vi "LakeShore Ramp Text In.vi"(1 "command text in":string[](array[string])=["N/A", "Magent PS", "N/A", "Set Field", "Set Field to 2.0000E+0 @ 0.0000T /min, no wait , extra 0 sec wait", "N/A", "N/A", "", "1", "0", "N/A", "2.000000", "0.000000", "N/A", "N/A", "N/A", "N/A", "N/A", "N/A", "N/A", "N/A", "N/A", "N/A", "N/A", "N/A", "N/A", "N/A", "N/A", "N/A", "N/A", "N/A", "N/A", "N/A", "N/A"]) -> (0 "LSRamp":T1={"VISA Resource Name"="", "extra wait"=0, "start (K/W)"=1e-09, "end (K/W)"=0.001, "Sweep Time (H:M:S)"=3600.0, "Mapping"=FALSE, "Parameter"=FALSE, "Loop"=FALSE} {"Sweep Time (H:M:S)" format="%<%H:%M:%S>t"; "extra wait" min=0; "start (K/W)" format="%#.7e"; "end (K/W)" format="%#.7e"})   [LabVIEW 2020]
uses:
  LSRamp.ctl
panel:
  # "LakeShore Ramp"
  # "Log"
  # "Start Temp(K)/Power(W)"
  # "Sweep Time (HH:MM:SS)"
  # "End Temp(K)/Power(W)"
  # "Linear"
  # "seconds"
  # "AND wait extra"
  # "Power"
  # "Temp"
  # "VISA Name"
  # "Loop 2"
  # "Loop 1"
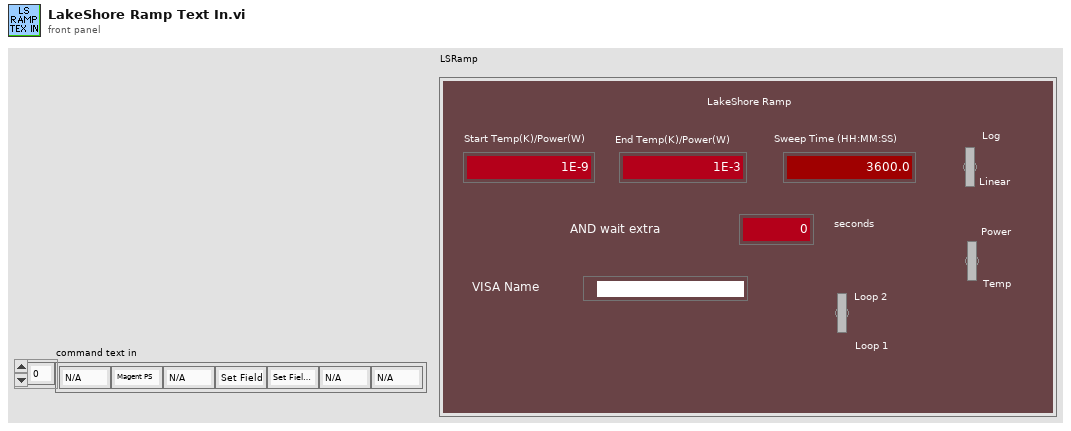
[diagram p1: front panel]
types:
  T1 = typedef "LSRamp.ctl" = cluster{"VISA Resource Name":refnum<visa-resource-name>, "extra wait":i32, "start (K/W)":dbl, "end (K/W)":dbl, "Sweep Time (H:M:S)":dbl, "Mapping":bool, "Parameter":bool, "Loop":bool}
  T2 = cluster{"command text in[0]":string, "command text in[1]":string, "command text in[2]":string, "command text in[3]":string, "command text in[4]":string, "command text in[5]":string, "command text in[6]":string, "command text in[7]":string, "command text in[8]":string, "command text in[9]":string, "command text in[10]":string, "command text in[11]":string, "command text in[12]":string, "command text in[13]":string, "command text in[14]":string, "command text in[15]":string, "command text in[16]":string, "command text in[17]":string, "command text in[18]":string, "command text in[19]":string}
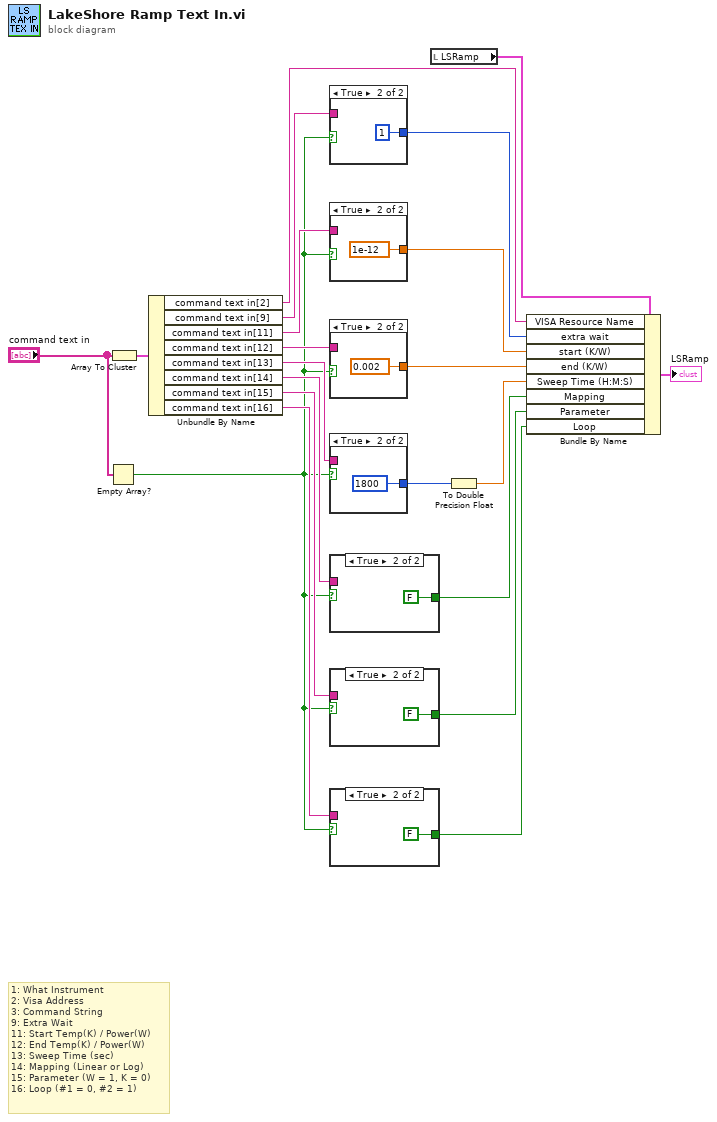
[diagram p0: block diagram]
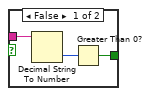
[diagram p2: hidden frame]
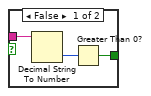
[diagram p3: hidden frame]
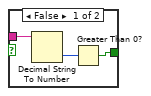
[diagram p4: hidden frame]
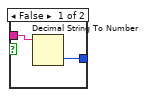
[diagram p5: hidden frame]
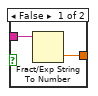
[diagram p6: hidden frame]
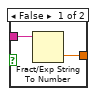
[diagram p7: hidden frame]
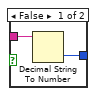
[diagram p8: hidden frame]
diagram:
  # "1: What Instrument\n2: Visa Address\n3: Command String\n9: Extra Wait\n11: Start Temp(K) / Power(W)\n12: End Temp(K) / Power(W)\n13: Sweep Time (sec)\n14: Mapping (Linear or Log)\n15: Parameter (W = 1, K = 0)\n16: Loop (#1 = 0, #2 = 1)"
  n1 = Empty Array?(array="command text in") -> (empty?=w3:bool)
  n2 = Array To Cluster(array="command text in") -> (cluster=w21:T2)
  n3 = Unbundle By Name(w21) -> ("command text in[2]"=w19:string, "command text in[9]"=w18:string, "command text in[11]"=w16:string, "command text in[12]"=w14:string, "command text in[13]"=w12:string, "command text in[14]"=w9:string, "command text in[15]"=w4:string, "command text in[16]"=w5:string)
  n4 = case shown="True" w3 {
    tunnel: w18 -> [w23 _]
    tunnel: [w22 u16 1 ("Value (Signaling)")] -> w17
    frame False {
      n5 = Decimal String To Number(string=w23) -> (number=w22:i32)  [unwired: 2 in, 1 out]
    }
    frame True {
    }
  }
  n6 = case shown="True" w3 {
    tunnel: [w26 1e-12] -> w15
    tunnel: w16 -> [w25 _]
    frame False {
      n7 = Fract/Exp String To Number(string=w25) -> (number=w26:dbl)  [unwired: 3 in, 1 out]
    }
    frame True {
    }
  }
  n8 = case shown="True" w3 {
    tunnel: [w29 0.002] -> w13
    tunnel: w14 -> [w28 _]
    frame False {
      n9 = Fract/Exp String To Number(string=w28) -> (number=w29:dbl)  [unwired: 3 in, 1 out]
    }
    frame True {
    }
  }
  n10 = case shown="True" w3 {
    tunnel: w12 -> [w32 _]
    tunnel: [w31 1800] -> w11
    frame False {
      n11 = Decimal String To Number(string=w32) -> (number=w31:i32)  [unwired: 2 in, 1 out]
    }
    frame True {
    }
  }
  n12 = case shown="True" w3 {
    tunnel: w9 -> [w36 _]
    tunnel: [w35 FALSE] -> w8
    frame False {
      n13 = Decimal String To Number(string=w36) -> (number=w34:i32)  [unwired: 2 in, 1 out]
      n14 = Greater Than 0?(x=w34) -> (x > 0?=w35:bool)
    }
    frame True {
    }
  }
  n15 = case shown="True" w3 {
    tunnel: w4 -> [w40 _]
    tunnel: [w39 FALSE] -> w2
    frame False {
      n16 = Decimal String To Number(string=w40) -> (number=w38:i32)  [unwired: 2 in, 1 out]
      n17 = Greater Than 0?(x=w38) -> (x > 0?=w39:bool)
    }
    frame True {
    }
  }
  n18 = case shown="True" w3 {
    tunnel: w5 -> [w44 _]
    tunnel: [w43 FALSE] -> w1
    frame False {
      n19 = Decimal String To Number(string=w44) -> (number=w42:i32)  [unwired: 2 in, 1 out]
      n20 = Greater Than 0?(x=w42) -> (x > 0?=w43:bool)
    }
    frame True {
    }
  }
  n21 = local read "LSRamp"() -> (w7:T1)
  n22 = To Double Precision Float(number=w11) -> (double precision float=w10:dbl)
  n23 = Bundle By Name(cluster=w7, "VISA Resource Name"=w19, "extra wait"=w17, "start (K/W)"=w15, "end (K/W)"=w13, "Sweep Time (H:M:S)"=w10, "Mapping"=w8, "Parameter"=w2, "Loop"=w1) -> (→"LSRamp":T1)
